vi "Page_Info_Read.vi"(6 "ctlReferences":T1, 8 "error in (no error)":errorcluster, 11 "AB_DepSourceDist in":refnum<class "AB_DepSourceDist.lvclass">) -> (0 "error out":errorcluster, 3 "AB_DepSourceDist out":refnum<class "AB_DepSourceDist.lvclass">)   [LabVIEW 2020, in "AB_DepSourceDist.lvclass"]
uses:
  <vilib>/AppBuilder/AB_Classes/DepSourceDist/AB_DepSourceDist.lvclass
  e:/builds/penguin/labview/branches/2020/dev/dist/vi.lib/AppBuilder/AB_Classes/Build/AB_Build.lvclass
  <resource>/Framework/Providers/Builds/AppBuilder/AB_UI_Page_Info_References.ctl
  <vilib>/AppBuilder/AB_Classes/SourceDistribution/AB_SourceDistribution.lvclass
  <vilib>/AppBuilder/AB_Classes/Deployment/AB_Deployment.lvlib
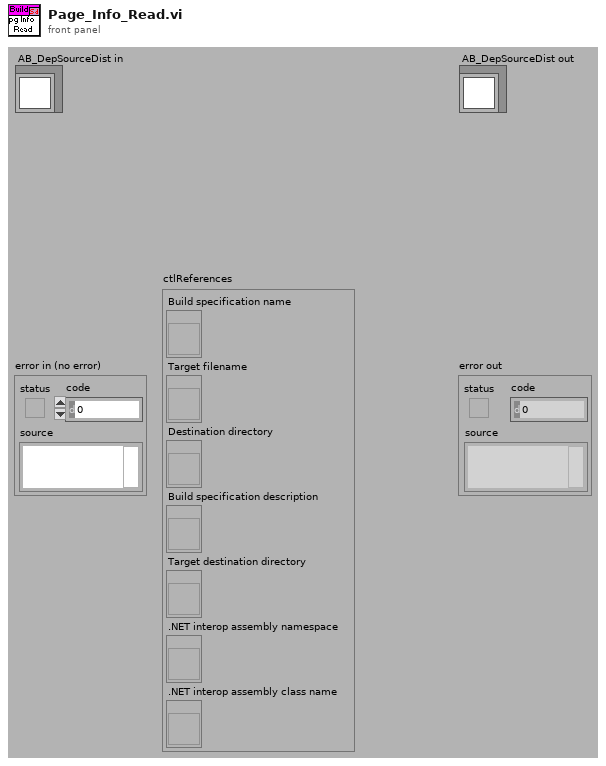
[diagram p1: front panel]
types:
  T1 = typedef "AB_UI_Page_Info_References.ctl" = cluster{"Build specification name":refnum<vi>, "Target filename":refnum<vi>, "Destination directory":refnum<vi>, "Build specification description":refnum<vi>, "Target destination directory":refnum<vi>, ".NET interop assembly namespace":refnum<vi>, ".NET interop assembly class name":refnum<vi>}
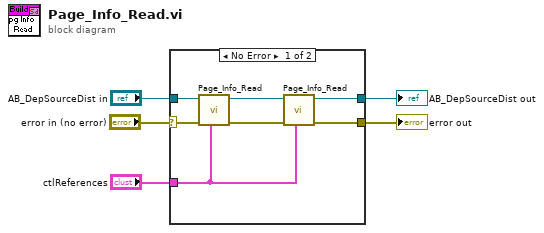
[diagram p0: block diagram]
diagram:
  n1 = case shown="No Error" "error in (no error)" {
    selector: "error in (no error)" -> [w12 w14]
    tunnel: [w8 w14] -> w3
    tunnel: "AB_DepSourceDist in" -> [w11 w13]
    tunnel: "ctlReferences" -> [w10 _]
    tunnel: [w6 w13] -> w4
    frame No Error {
      n2 = call-parent <vilib>:"Page_Info_Read.vi"("ctlReferences"=w10, "error in (no error)"=w12, "AB_Build in"=w11) -> ("error out"=w9:errorcluster, "AB_Build out"=w7:refnum<class "AB_DepSourceDist.lvclass">)  [unwired: 7 in]
      n3 = call <vilib>:"Page_Info_Read.vi"("ctlReferences"=w10, "error in (no error)"=w9, "Build in"=w7) -> ("error out"=w8:errorcluster, "Build out"=w6:refnum<class "AB_DepSourceDist.lvclass">)  [unwired: 7 in]
    }
    frame Error {
    }
  }
  "error out" <- w3
  "AB_DepSourceDist out" <- w4
